vi "Build Methods.vi"(8 "error in (no error)":errorcluster, 9 "Wiring Spec":T1, 11 "CS++Actor in":refnum<class "CS++Actor.lvclass">) -> (0 "error out":errorcluster, 3 "CS++Actor out":refnum<class "CS++Actor.lvclass">)   [LabVIEW 2014, in "CS++Actor.lvlib" / "CS++Actor.lvclass"]
doc: "Creates the methods for the new message."
uses:
  CS++Actor.lvclass
  CS++Actor.lvclass/CS++Actor.ctl
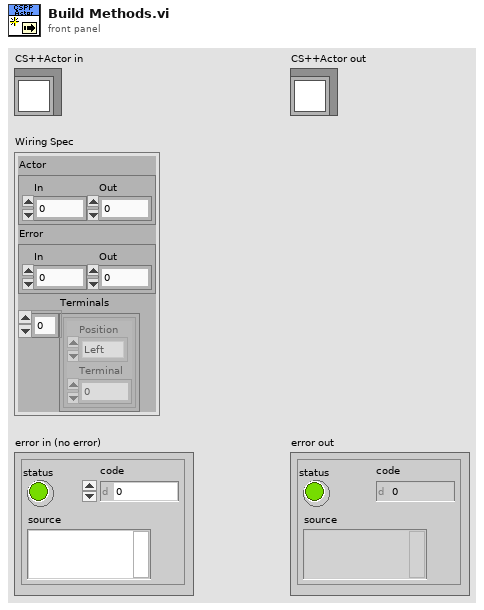
[diagram p1: front panel]
types:
  T1 = cluster{"Actor":cluster{"In":i32, "Out":i32}, "Error":cluster{"In":i32, "Out":i32}, "Terminals":cluster{"Position":enum16{"Left", "Top", "Bottom", "Right"}, "Terminal":i32}[]}
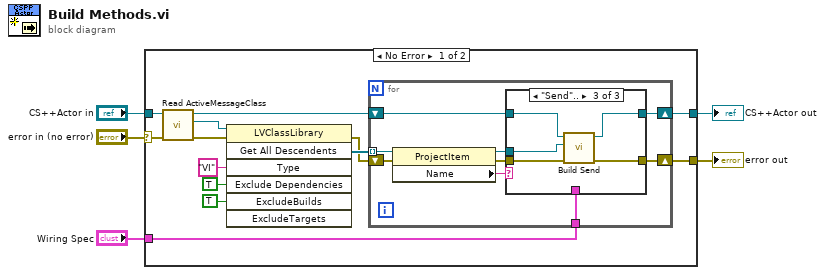
[diagram p0: block diagram]
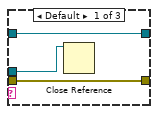
[diagram p2: hidden frame]
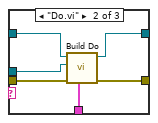
[diagram p3: hidden frame]
diagram:
  n1 = case shown="No Error" "error in (no error)" {
    selector: "error in (no error)" -> [w8 w43]
    tunnel: [w13 w43] -> w4
    tunnel: [w11 w42] -> w2
    tunnel: "CS++Actor in" -> [w9 w42]
    tunnel: "Wiring Spec" -> [w12 _]
    frame No Error {
      n2 = call "Read ActiveMessageClass.vi"("error in (no error)"=w8, "CS++Actor in"=w9) -> ("error out"=w6:errorcluster, "ActiveMessageClass"=w10:refnum<vi>, "CS++Actor out"=w7:refnum<class "CS++Actor.lvclass">)  [unwired: 7 in]
      n3 = invoke class="LVClassLibrary" method="Get All Descendents"(reference=w10, error in=w6, "Type"="VI", "Exclude Dependencies"=TRUE ("ExcludeDependencies"), "ExcludeBuilds"=TRUE) -> (error out=w14:errorcluster, "All Descendents"=w15:refnum<vi>[])  [unwired: 2 in, 5 out]
      n4 = for {
        tunnel: w15 -> [w27] mode=indexing
        shift-right: [w24] -> w13
        shift-left: w14 -> [w26]
        tunnel: w12 -> [w21]
        shift-right: [w19] -> w11
        shift-left: w7 -> [w20]
        n5 = property class="ProjectItem"(reference=w27, error in=w26) -> (reference out=w22:refnum<vi>, error out=w23:errorcluster, "Name"=w25:string)
        n6 = case shown="\"Send\".." w25 {
          tunnel: [w30 w35 w40] -> w24
          tunnel: w23 -> [w30 w36 w41]
          tunnel: w22 -> [w29 w33 w37]
          tunnel: w21 -> [_ w34 _]
          tunnel: w20 -> [w28 w32 w39]
          tunnel: [w28 w31 w38] -> w19
          frame Default {
            n7 = Close Reference(reference=w29) -> ()  [unwired: 1 in, 1 out]
          }
          frame "Do.vi" {
            n8 = call "Build Do.vi"("Wiring Spec"=w34, "error in (no error)"=w36, "Do VI"=w33, "CS++Actor in"=w32) -> ("error out"=w35:errorcluster, "CS++Actor out"=w31:refnum<class "CS++Actor.lvclass">)  [unwired: 6 in]
          }
          frame "Send".. {
            n9 = call "Build Send.vi"("error in (no error)"=w41, "Send VI"=w37, "CS++Actor in"=w39) -> ("error out"=w40:errorcluster, "CS++Actor out"=w38:refnum<class "CS++Actor.lvclass">)  [unwired: 7 in]
          }
        }
      }
    }
    frame Error {
    }
  }
  "error out" <- w4
  "CS++Actor out" <- w2
